vi "Scroll Gradient With Timer.vi"(8 "error in (no error)":errorcluster caption="错误输入（无错误）", 10 "Time Target (s)":dbl=0.05 caption="目标时间(s)", 11 "Scroll Gradient 输入":refnum<class "Scroll Gradient.lvclass"> caption="DNL_LabVIEW Object in") -> (0 "error out":errorcluster caption="错误输出", 3 "Scroll Gradient 输出":refnum<class "Scroll Gradient.lvclass"> caption="DNL_LabVIEW Object out")   [LabVIEW 2012, in "Picture Box Tools.lvlib" / "Scroll Gradient.lvclass"]
uses:
  Scroll Gradient.lvclass
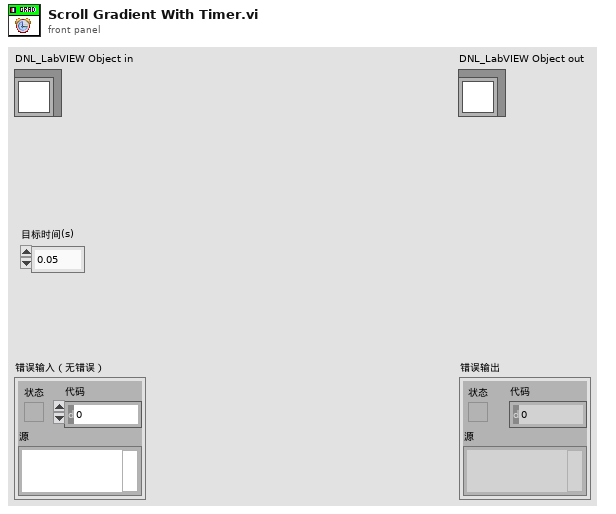
[diagram p1: front panel]
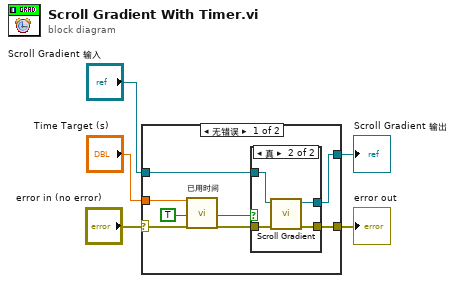
[diagram p0: block diagram]
diagram:
  n1 = case shown="无错误" "error in (no error)" {
    selector: "error in (no error)" -> [w10 w21]
    tunnel: [w6 w21] -> w4
    tunnel: [w11 w20] -> w2
    tunnel: "Scroll Gradient 输入" -> [w7 w20]
    tunnel: "Time Target (s)" -> [w13 _]
    frame No Error {
      n2 = call "已用时间"("Time Target (s)"=w13, "Auto Reset"=TRUE, "error in (no error)"=w10) -> ("Time has Elapsed"=w8:bool, "error out"=w9:errorcluster)  [unwired: 9 in, 6 out]
      n3 = case shown="真" w8 {
        tunnel: [w15 w19] -> w11
        tunnel: w9 -> [w14 w18]
        tunnel: w7 -> [w15 w17]
        tunnel: [w14 w16] -> w6
        frame False {
        }
        frame True {
          n4 = call "Scroll Gradient.vi"("error in (no error)"=w18, "Scroll Gradient 输入"=w17) -> ("error out"=w16:errorcluster, "Scroll Gradient 输出"=w19:refnum<class "Scroll Gradient.lvclass">)  [unwired: 8 in]
        }
      }
    }
    frame Error {
    }
  }
  "error out" <- w4
  "Scroll Gradient 输出" <- w2
